vi "Teleop.vi"(10 "Match Info":T2={"Autonomous Elapsed Seconds"=0.0, "TeleOp Elapsed Seconds"=0.0, "Disabled Elapsed Seconds"=0.0, "Visited Autonomous"=FALSE, "Visited TeleOp"=FALSE, "Visited Disabled"=FALSE, "Autonomous Settings"={"Autonomous Style"=enum."Independent", "VI Refnum"=refnum}}, 11 "Call Context":T3) -> ()   [LabVIEW 2017]
doc: "This VI is called for each TeleOp packet received from the DS where the robot is not disabled. It is often used to read from the joysticks and update I/O or to update setpoints for timed control loops. It should complete and return within 20 milliseconds or it may miss DS packets."
uses:
  <vilib>/Rock Robotics/WPI/DriverStation/WPI_DriverStationDerivedRobotMode.ctl
  <vilib>/Rock Robotics/WPI/DriverStation/WPI_DriverStationMatch Info.ctl
  <vilib>/Rock Robotics/Network Tables/NT Read Boolean.vi
  <vilib>/Rock Robotics/Network Tables/NT Read Number.vi
  <vilib>/Rock Robotics/WPI/Utilities/WPI_GetSetVariantRefNum.vi
  <vilib>/Rock Robotics/Network Tables/NT Write Numeric Array.vi
  <vilib>/Rock Robotics/Network Tables/NT Write Boolean Array.vi
panel:
  in  "Bbutton":T1(array[cluster])=[{"Movement"="Pause", "Delay (sec)"=1.0, "X Joystick Value"=0.0, "Y Joystick Value"=0.0}, {"Movement"="Forward 90 in", "Delay (sec)"=1.0, "X Joystick Value"=0.0, "Y Joystick Value"=0.8}, {"Movement"="Puase", "Delay (sec)"=1.0, "X Joystick Value"=0.0, "Y Joystick Value"=0.0}, {"Movement"="Pause\nForward 60 in", "Delay (sec)"=1.0, "X Joystick Value"=0.0, "Y Joystick Value"=0.0}, {"Movement"="Pause", "Delay (sec)"=1.0, "X Joystick Value"=0.0, "Y Joystick Value"=0.0}, {"Movement"="Pause", "Delay (sec)"=1.0, "X Joystick Value"=0.0, "Y Joystick Value"=0.0}]
  in  "Xbutton":T1(array[cluster])=[{"Movement"="Pause", "Delay (sec)"=1.0, "X Joystick Value"=0.0, "Y Joystick Value"=0.0}, {"Movement"="Forward 90 in", "Delay (sec)"=1.0, "X Joystick Value"=0.0, "Y Joystick Value"=0.85}, {"Movement"="Puase", "Delay (sec)"=1.0, "X Joystick Value"=0.0, "Y Joystick Value"=0.0}, {"Movement"="Forward 60\nForward 60 in", "Delay (sec)"=1.0, "X Joystick Value"=0.0, "Y Joystick Value"=0.0}, {"Movement"="Forward 90 in", "Delay (sec)"=1.0, "X Joystick Value"=0.0, "Y Joystick Value"=0.0}, {"Movement"="Forward 90 in", "Delay (sec)"=1.0, "X Joystick Value"=0.0, "Y Joystick Value"=0.0}]
  out "Sample Slider 0":dbl(slide) scale=0.0..5.0
  out "Sample Boolean 1":bool
  out "Sample Boolean 0":bool
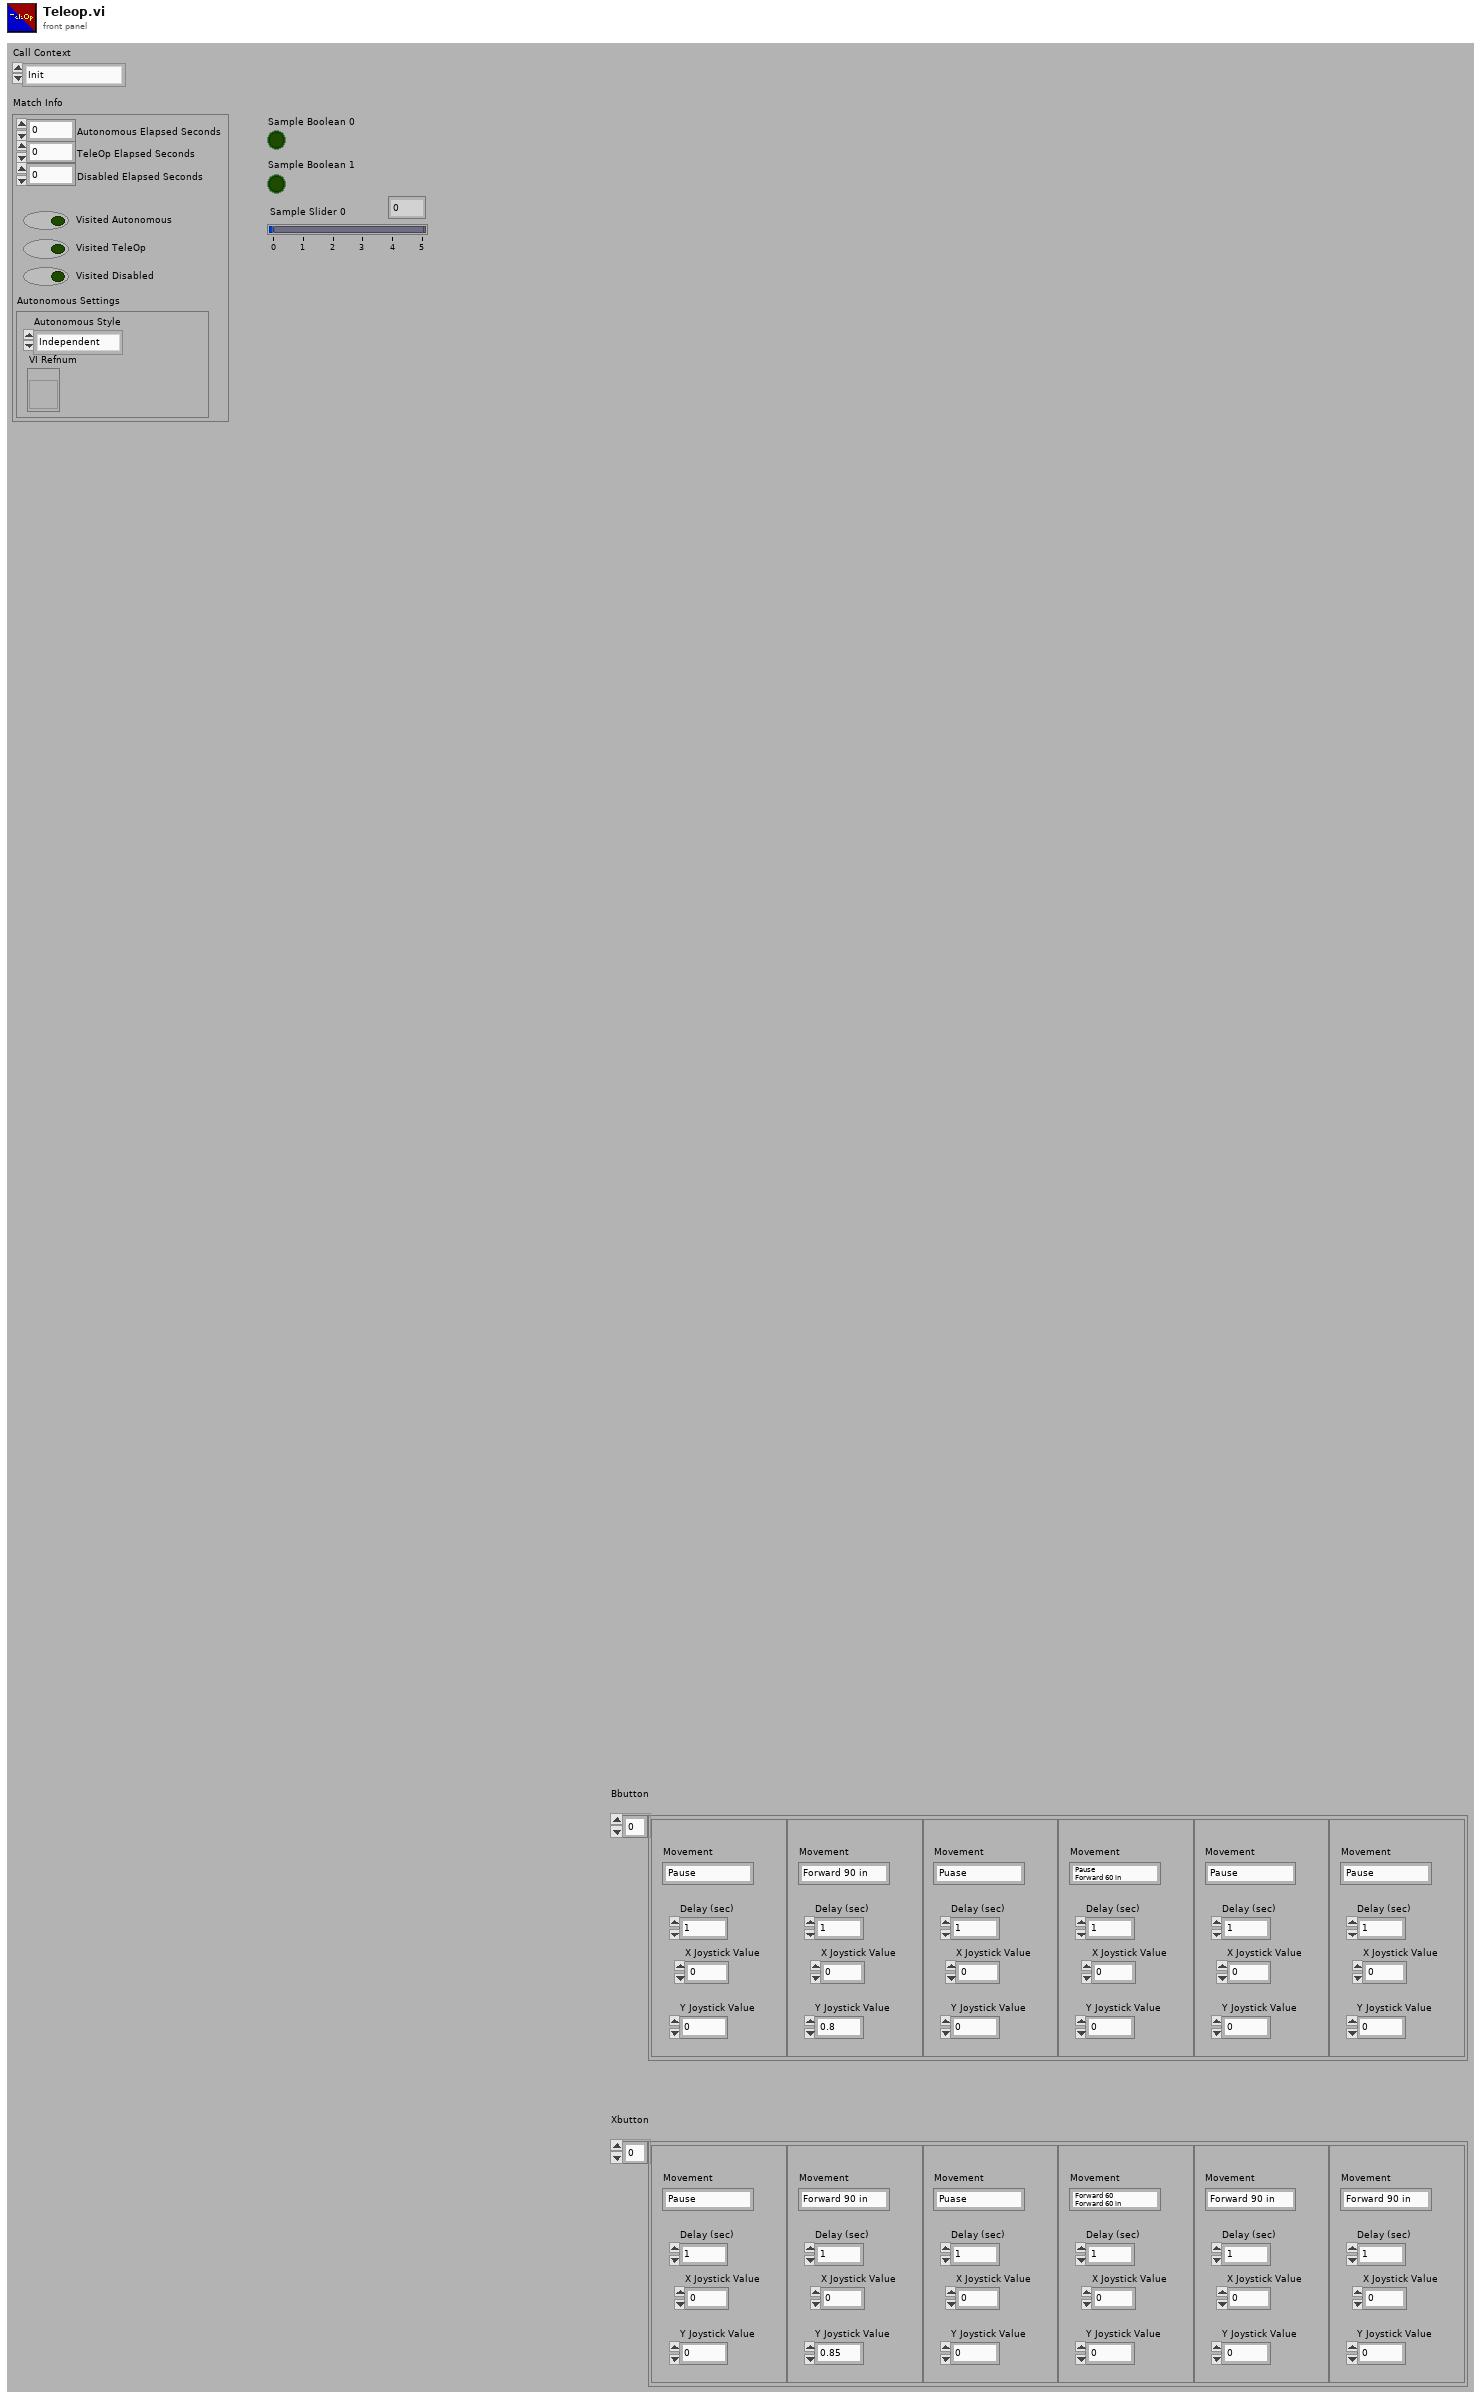
[diagram p1: front panel]
types:
  T1 = cluster{"Movement":string, "Delay (sec)":dbl, "X Joystick Value":dbl, "Y Joystick Value":dbl}[]
  T2 = typedef "WPI_DriverStationMatch Info.ctl" = cluster{"Autonomous Elapsed Seconds":dbl, "TeleOp Elapsed Seconds":dbl, "Disabled Elapsed Seconds":dbl, "Visited Autonomous":bool, "Visited TeleOp":bool, "Visited Disabled":bool, "Autonomous Settings":cluster{"Autonomous Style":enum16{"Iterative", "Independent"}, "VI Refnum":refnum<vi>}}
  T3 = typedef "WPI_DriverStationDerivedRobotMode.ctl" = enum16{"Init", "Execute", "Stop"}
  T4 = typedef "WPI_RobotDriveDevRef.ctl" = cluster{"DevStatus":errorcluster, "Motors[]":T5[], "Square Inputs":bool, "Max Output":dbl}
  T5 = typedef "WPI_MotorControlDeviceRef.ctl" = cluster{"DeviceStatus":errorcluster, "Type":T6, "PWM":cluster{"PWM Channel":T7, "DeadBand":T8}, "CAN":cluster{"Device Number":u8, "SetOutput VI Ref":variant, "GetOutput VI Ref":variant, "Enable VI Ref":variant, "Disable VI Ref":variant, "Data":variant}, "Invert":bool, "DIO PWM":cluster{"PWM \"Enable\" Channel":T7, "DIOChannel":T9, "PWM Rate":dbl}}
  T6 = typedef "WPI_MotorControlType.ctl" = enum16{"PWM", "CAN", "DIO PWM"}
  T7 = typedef "FPGA_DIOPWMChannel.ctl" = enum8{"PWM 0", "PWM 1", "PWM 2", "PWM 3", "PWM 4", "PWM 5", "PWM 6", "PWM 7", "PWM 8", "PWM 9", "PWM MXP 0", "PWM MXP 1", "PWM MXP 2", "PWM MXP 3", "PWM MXP 4", "PWM MXP 5", "PWM MXP 6", "PWM MXP 7", "PWM MXP 8", "PWM MXP 9", "Invalid"}
  T8 = typedef "WPI_PWMDeadband.ctl" = cluster{"Name":string, "maxPositivePwm":i32, "minPositivePwm":i32, "centerPwm":i32, "maxNegativePwm":i32, "minNegativePwm":i32, "angularRange":u16}
  T9 = typedef "FPGA_DIOChannel.ctl" = enum8{"DIO 0", "DIO 1", "DIO 2", "DIO 3", "DIO 4", "DIO 5", "DIO 6", "DIO 7", "DIO 8", "DIO 9", "DIO MXP 0", "DIO MXP 1", "DIO MXP 2", "DIO MXP 3", "DIO MXP 4", "DIO MXP 5", "DIO MXP 6", "DIO MXP 7", "DIO MXP 8", "DIO MXP 9", "DIO MXP 10", "DIO MXP 11", "DIO MXP 12", "DIO MXP 13", "DIO MXP 14", "DIO MXP 15", "SPI Port CS1", "SPI Port CS2", "SPI Port CS3", "SPI Port MISO", "SPI Port MOSI", "Invalid"}
  T10 = typedef "WPI_JoystickDevRef.ctl" = cluster{"Device":T11}
  T11 = typedef "WPI_JoystickDeviceEnum.ctl" = enum16{"USB 0", "USB 1", "USB 2", "USB 3", "USB 4", "USB 5"}
  T12 = cluster{"Axes[0]":dbl, "Axes[1]":dbl, "Axes[2]":dbl, "Axes[3]":dbl, "Axes[4]":dbl, "Axes[5]":dbl, "Axes[6]":dbl, "Axes[7]":dbl, "Axes[8]":dbl}
  T13 = cluster{"Buttons[0]":bool, "Buttons[1]":bool, "Buttons[2]":bool, "Buttons[3]":bool, "Buttons[4]":bool, "Buttons[5]":bool, "Buttons[6]":bool, "Buttons[7]":bool, "Buttons[8]":bool}
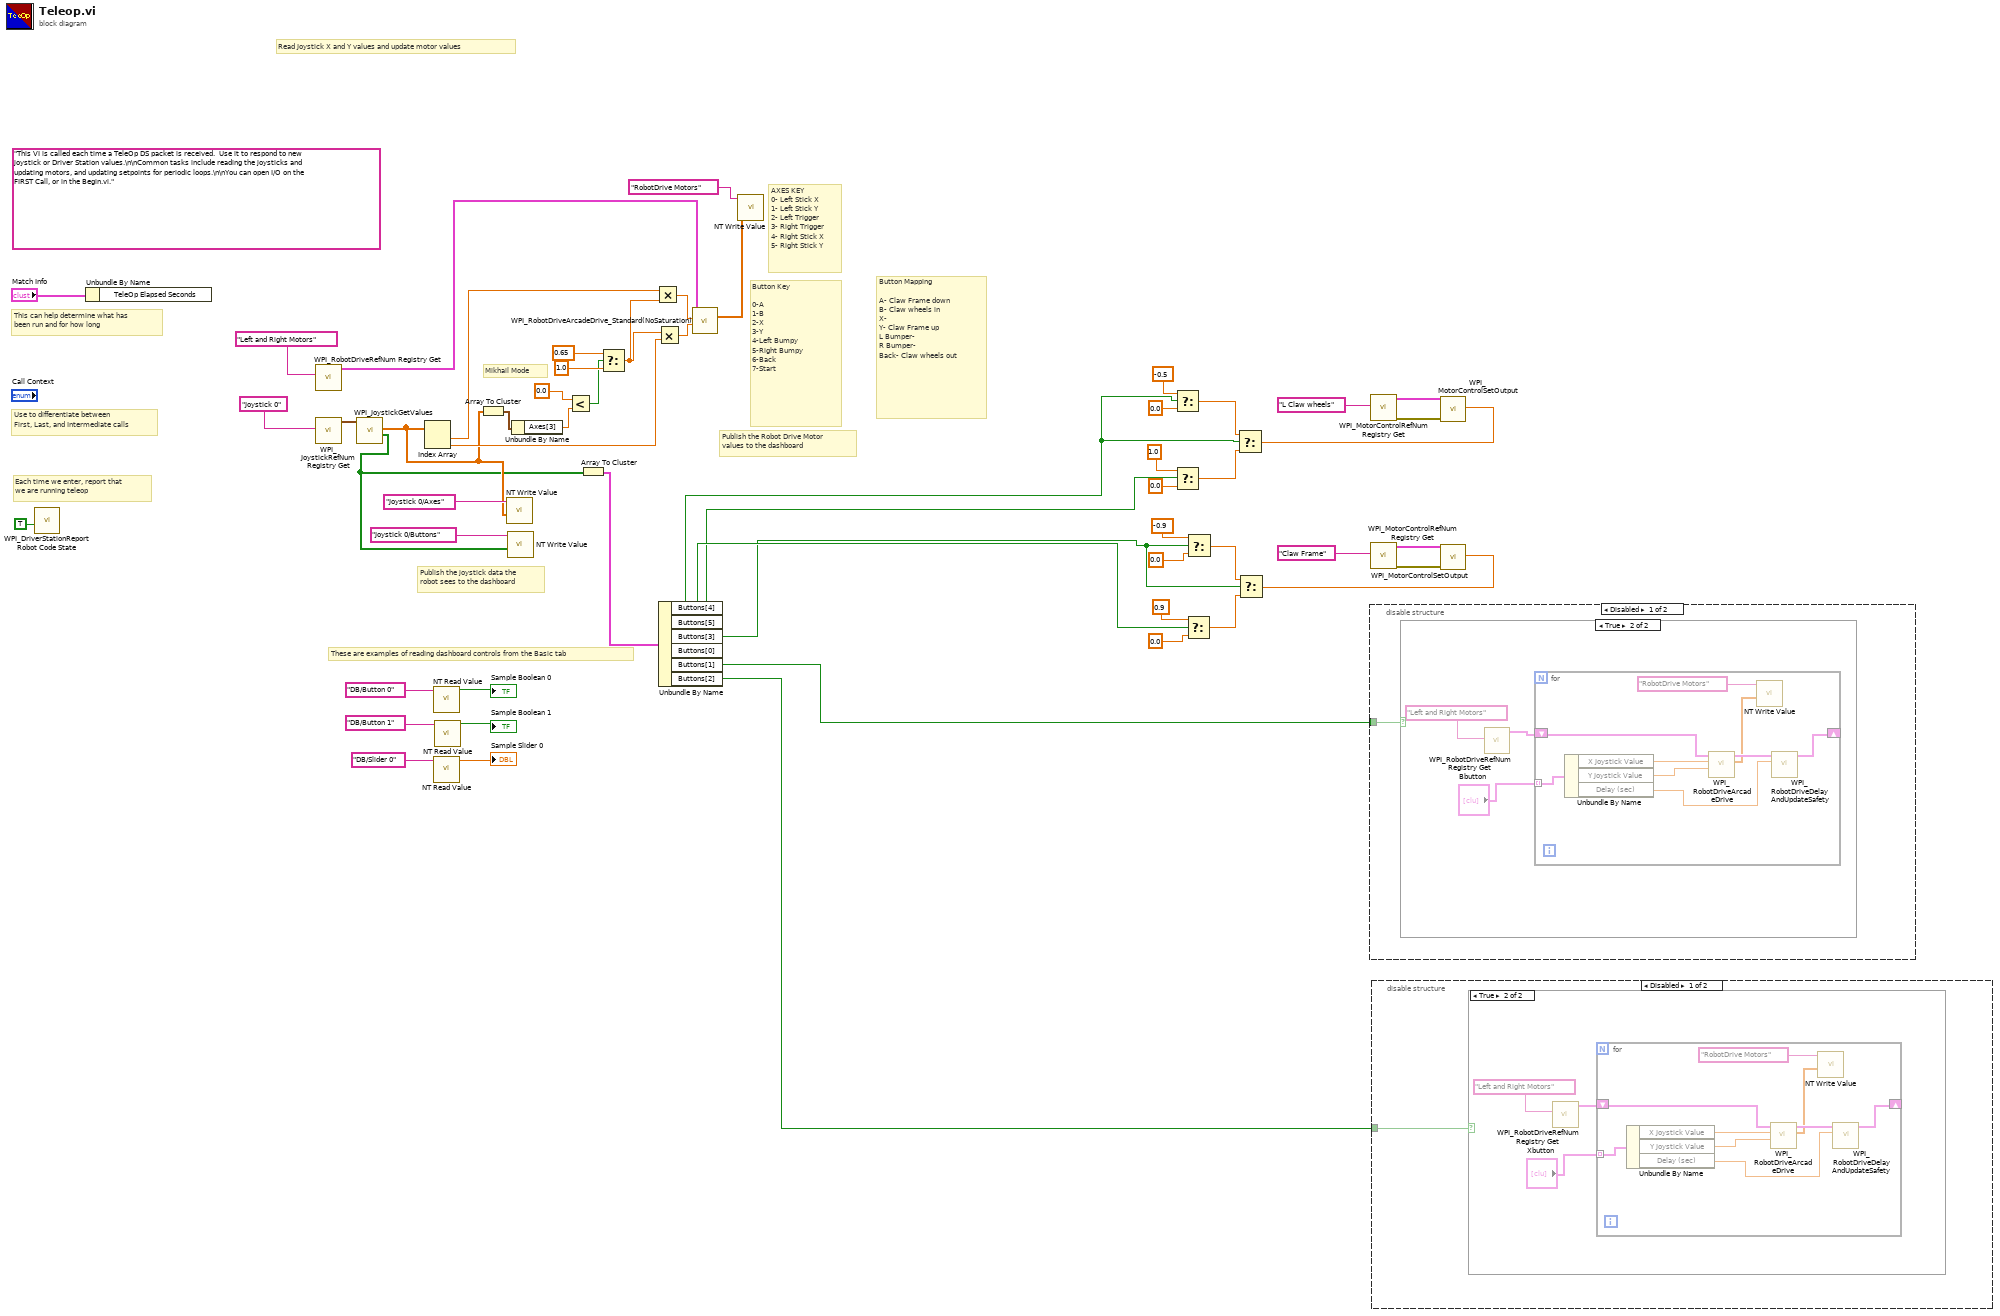
[diagram p0: block diagram]
diagram:
  (unwired) "This VI is called each time a TeleOp DS packet is received.  Use it to respond to new joystick or Driver Station values.\n\nCommon tasks include reading the joysticks and updating motors, and updating setpoints for periodic loops.\n\nYou can open I/O on the FIRST Call, or in the Begin.vi."
  # "AXES KEY\n0- Left Stick X\n1- Left Stick Y\n2- Left Trigger\n3- Right Trigger\n4- Right Stick X\n5- Right Stick Y"
  # "Mikhail Mode"
  # "Button Mapping\n\nA- Claw Frame down\nB- Claw wheels in\nX- \nY- Claw Frame up\nL Bumper-\nR Bumper-\nBack- Claw wheels out"
  # "Button Key\n\n0-A\n1-B\n2-X\n3-Y\n4-Left Bumpy\n5-Right Bumpy\n6-Back\n7-Start"
  # "These are examples of reading dashboard controls from the Basic tab"
  # "Publish the Robot Drive Motor\nvalues to the dashboard"
  # "Publish the joystick data the\nrobot sees to the dashboard"
  # "Each time we enter, report that\nwe are running teleop"
  # "Use to differentiate between\nFirst, Last, and Intermediate calls"
  # "This can help determine what has\nbeen run and for how long"
  # "Read Joystick X and Y values and update motor values"
  n1 = call <vilib>:"WPI_DriverStationReport Robot Code State.vi"("TeleOp"=TRUE ("Autonomous")) -> ()  [unwired: 10 in, 1 out]
  n2 = Unbundle By Name("Match Info") -> ()  [unwired: 1 out]
  n3 = call <vilib>:"WPI_RobotDriveRefNum Registry Get.vi"("refnum name"="Left and Right Motors") -> ("RobotDriveDevRef"=w19:T4)  [unwired: 1 in, 9 out]
  n4 = call <vilib>:"WPI_JoystickRefNum Registry Get.vi"("refnum name"="Joystick 0") -> ("JoystickDevRef"=w17:T10)  [unwired: 1 in, 9 out]
  n5 = call <vilib>:"WPI_JoystickGetValues.vi"("JoystickDevRef"=w17) -> ("Buttons"=w7:bool[], "Axes"=w8:dbl[])  [unwired: 6 in, 3 out]
  n6 = Index Array(array=w8) -> (element #1=w6:dbl, element #2=w9:dbl)  [unwired: 2 in]
  n7 = call-poly <vilib>:"NT Read Value.vi"("Name"="DB/Button 0" ("refnum name")) -> ("Boolean"=→"Sample Boolean 0":bool)  [unwired: 9 in, 1 out]
  n8 = call-poly <vilib>:"NT Read Value.vi"("Name"="DB/Slider 0" ("refnum name")) -> ("Numeric"=→"Sample Slider 0":dbl)  [unwired: 9 in, 1 out]
  n9 = call-poly <vilib>:"NT Read Value.vi"("Name"="DB/Button 1" ("refnum name")) -> ("Boolean"=→"Sample Boolean 1":bool)  [unwired: 9 in, 1 out]
  n10 = Array To Cluster(array=w8) -> (cluster=w14:T12)
  n11 = call-poly <vilib>:"NT Write Value.vi"("Numeric Array"=w8, "Name"="Joystick 0/Axes") -> ()  [unwired: 9 in, 1 out]
  n12 = call-poly <vilib>:"NT Write Value.vi"("Boolean Array"=w7, "Name"="Joystick 0/Buttons") -> ()  [unwired: 9 in, 1 out]
  n13 = Unbundle By Name(w14) -> ("Axes[3]"=w2:dbl)
  n14 = Less?(x=0.0, y=w2) -> (x < y?=w1:bool)
  n15 = Array To Cluster(array=w7) -> (cluster=w23:T13)
  n16 = Select(t=0.65, s=w1, f=1.0) -> (s? t:f=w5:dbl)
  n17 = Multiply(x=w6, y=w5) -> (x*y=w4:dbl)
  n18 = Multiply(x=w5, y=w9) -> (x*y=w10:dbl)
  n19 = Unbundle By Name(w23) -> ("Buttons[4]"=w28:bool, "Buttons[5]"=w3:bool, "Buttons[3]"=w25:bool, "Buttons[0]"=w32:bool, "Buttons[1]"=w21:bool, "Buttons[2]"=w22:bool)
  n20 = call <vilib>:"WPI_RobotDriveArcadeDrive_Standard(NoSaturation).vi"("Y axis value"=w10, "X axis value"=w4, "RobotDriveDevRef"=w19) -> ("Motor Values"=w16:dbl[])  [unwired: 1 in, 7 out]
  n21 = call-poly <vilib>:"NT Write Value.vi"("Numeric Array"=w16, "Name"="RobotDrive Motors") -> ()  [unwired: 9 in, 1 out]
  n22 = Select(t=-0.5, s=w28, f=0.0) -> (s? t:f=w31:dbl)
  n23 = Select(t=1.0, s=w3, f=0.0) -> (s? t:f=w30:dbl)
  n24 = Select(t=0.9, s=w32, f=0.0) -> (s? t:f=w26:dbl)
  n25 = Select(t=-0.9, s=w25, f=0.0) -> (s? t:f=w27:dbl)
  n26 = Select(t=w31, s=w28, f=w30) -> (s? t:f=w29:dbl)
  n27 = Select(t=w27, s=w25, f=w26) -> (s? t:f=w24:dbl)
  n28 = disable-structure shown="Disabled" {
    disable-tunnel: w21 -> [w57 _]
    frame Disabled {
      n29 = case shown="True" w57 {
        frame False {
        }
        frame True {
          n30 = call <vilib>:"WPI_RobotDriveRefNum Registry Get.vi"("refnum name"="Left and Right Motors") -> ("RobotDriveDevRef"=w59:T4)  [unwired: 1 in, 9 out]
          n31 = for {
            shift-right: [w67] -> _
            shift-left: w59 -> [w68]
            tunnel: "Bbutton" -> [w63] mode=indexing
            n32 = Unbundle By Name(w63) -> ("X Joystick Value"=w66:dbl, "Y Joystick Value"=w65:dbl, "Delay (sec)"=w64:dbl)
            n33 = call-poly <vilib>:"WPI_RobotDriveArcadeDrive.vi"("Y axis value"=w65, "X axis value"=w66, "RobotDriveDevRef"=w68) -> ("Motor Values"=w61:dbl[], "RobotDriveDevRef"=w69:T4)  [unwired: 1 in, 6 out]
            n34 = call-poly <vilib>:"NT Write Value.vi"("Numeric Array"=w61, "Name"="RobotDrive Motors") -> ()  [unwired: 9 in, 1 out]
            n35 = call <vilib>:"WPI_RobotDriveDelayAndUpdateSafety.vi"("Delay (s)"=w64, "RobotDriveDevRef"=w69) -> ("RobotDriveDevRef 2"=w67:T4)  [unwired: 8 in, 1 out]
          }
        }
      }
    }
    frame Enabled {
    }
  }
  n36 = call <vilib>:"WPI_MotorControlRefNum Registry Get.vi"("refnum name"="L Claw wheels") -> ("error out"=w35:errorcluster, "MotorControlDevRef"=w34:T5)  [unwired: 9 in]
  n37 = call <vilib>:"WPI_MotorControlRefNum Registry Get.vi"("refnum name"="Claw Frame") -> ("error out"=w40:errorcluster, "MotorControlDevRef"=w39:T5)  [unwired: 9 in]
  n38 = disable-structure shown="Disabled" {
    disable-tunnel: w22 -> [w70 _]
    frame Disabled {
      n39 = case shown="True" w70 {
        frame False {
        }
        frame True {
          n40 = call <vilib>:"WPI_RobotDriveRefNum Registry Get.vi"("refnum name"="Left and Right Motors") -> ("RobotDriveDevRef"=w72:T4)  [unwired: 1 in, 9 out]
          n41 = for {
            shift-right: [w80] -> _
            shift-left: w72 -> [w81]
            tunnel: "Xbutton" -> [w76] mode=indexing
            n42 = Unbundle By Name(w76) -> ("X Joystick Value"=w79:dbl, "Y Joystick Value"=w78:dbl, "Delay (sec)"=w77:dbl)
            n43 = call-poly <vilib>:"WPI_RobotDriveArcadeDrive.vi"("Y axis value"=w78, "X axis value"=w79, "RobotDriveDevRef"=w81) -> ("Motor Values"=w74:dbl[], "RobotDriveDevRef"=w82:T4)  [unwired: 1 in, 6 out]
            n44 = call-poly <vilib>:"NT Write Value.vi"("Numeric Array"=w74, "Name"="RobotDrive Motors") -> ()  [unwired: 9 in, 1 out]
            n45 = call <vilib>:"WPI_RobotDriveDelayAndUpdateSafety.vi"("Delay (s)"=w77, "RobotDriveDevRef"=w82) -> ("RobotDriveDevRef 2"=w80:T4)  [unwired: 8 in, 1 out]
          }
        }
      }
    }
    frame Enabled {
    }
  }
  n46 = call <vilib>:"WPI_MotorControlSetOutput.vi"("error in (no error)"=w35, "Output"=w29, "MotorControlDevRef"=w34) -> ()  [unwired: 6 in, 3 out]
  n47 = call <vilib>:"WPI_MotorControlSetOutput.vi"("error in (no error)"=w40, "Output"=w24, "MotorControlDevRef"=w39) -> ()  [unwired: 6 in, 3 out]
